vi "Switch Channel.vi"(4 "error in (no error)":errorcluster, 5 "Channel to select":T1(ring), 6 "Card Number":u8=1 min=1 max=5 step=1, 7 "VISA resource in":refnum<visa-resource-name>) -> (0 "error out":errorcluster, 3 "VISA resource out":refnum<visa-resource-name>)   [LabVIEW 2015]
doc: "Switch the multiplexer in the selected card slot to the chosen channel. Designed for use with the HP3488A Switch Unit (5 slots) and the 44476A cards (4 channels)."
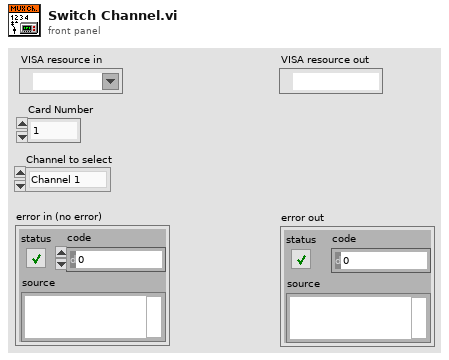
[diagram p1: front panel]
types:
  T1 = enum16{"Channel 1", "Channel 2", "Channel 3", "Channel 4"}
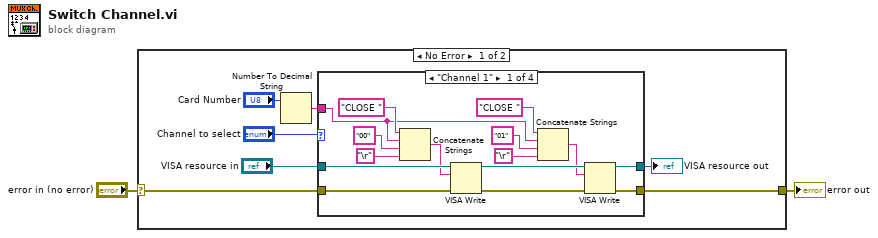
[diagram p0: block diagram]
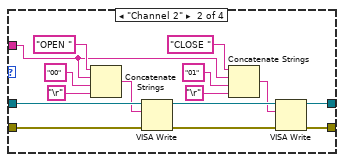
[diagram p2: hidden frame]
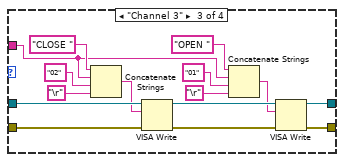
[diagram p3: hidden frame]
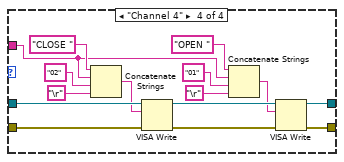
[diagram p4: hidden frame]
diagram:
  n1 = case shown="No Error" "error in (no error)" {
    selector: "error in (no error)" -> [w3 w70]
    tunnel: [w6 w70] -> w2
    frame No Error {
      n2 = Number To Decimal String(number="Card Number") -> (decimal integer string=w4:string)  [unwired: 1 in]
      n3 = case shown="\"Channel 1\"" "Channel to select" {
        tunnel: "VISA resource in" -> [w24 w39 w54 w69]
        tunnel: w3 -> [w23 w38 w53 w68]
        tunnel: [w20 w35 w50 w65] -> w7
        tunnel: [w19 w34 w49 w64] -> w6
        tunnel: w4 -> [w11 w26 w41 w56]
        frame "Channel 1" {
          n4 = Concatenate Strings("CLOSE " ("string"), w11, "00" ("write buffer"), "\r") -> (w16:string)
          n5 = VISA Write(VISA resource name=w24, write buffer=w16, error in (no error)=w23) -> (VISA resource name out=w22:refnum<visa-resource-name>, error out=w21:errorcluster)  [unwired: 1 out]
          n6 = Concatenate Strings("CLOSE " ("string"), w11, "01" ("write buffer"), "\r") -> (w10:string)
          n7 = VISA Write(VISA resource name=w22, write buffer=w10, error in (no error)=w21) -> (VISA resource name out=w20:refnum<visa-resource-name>, error out=w19:errorcluster)  [unwired: 1 out]
        }
        frame "Channel 2" {
          n8 = Concatenate Strings("OPEN " ("string"), w26, "00" ("write buffer"), "\r") -> (w31:string)
          n9 = VISA Write(VISA resource name=w39, write buffer=w31, error in (no error)=w38) -> (VISA resource name out=w37:refnum<visa-resource-name>, error out=w36:errorcluster)  [unwired: 1 out]
          n10 = Concatenate Strings("CLOSE " ("string"), w26, "01" ("write buffer"), "\r") -> (w25:string)
          n11 = VISA Write(VISA resource name=w37, write buffer=w25, error in (no error)=w36) -> (VISA resource name out=w35:refnum<visa-resource-name>, error out=w34:errorcluster)  [unwired: 1 out]
        }
        frame "Channel 3" {
          n12 = Concatenate Strings("CLOSE " ("string"), w41, "02" ("write buffer"), "\r") -> (w46:string)
          n13 = VISA Write(VISA resource name=w54, write buffer=w46, error in (no error)=w53) -> (VISA resource name out=w52:refnum<visa-resource-name>, error out=w51:errorcluster)  [unwired: 1 out]
          n14 = Concatenate Strings("OPEN " ("string"), w41, "01" ("write buffer"), "\r") -> (w40:string)
          n15 = VISA Write(VISA resource name=w52, write buffer=w40, error in (no error)=w51) -> (VISA resource name out=w50:refnum<visa-resource-name>, error out=w49:errorcluster)  [unwired: 1 out]
        }
        frame "Channel 4" {
          n16 = Concatenate Strings("CLOSE " ("string"), w56, "02" ("write buffer"), "\r") -> (w61:string)
          n17 = VISA Write(VISA resource name=w69, write buffer=w61, error in (no error)=w68) -> (VISA resource name out=w67:refnum<visa-resource-name>, error out=w66:errorcluster)  [unwired: 1 out]
          n18 = Concatenate Strings("OPEN " ("string"), w56, "01" ("write buffer"), "\r") -> (w55:string)
          n19 = VISA Write(VISA resource name=w67, write buffer=w55, error in (no error)=w66) -> (VISA resource name out=w65:refnum<visa-resource-name>, error out=w64:errorcluster)  [unwired: 1 out]
        }
      }
      "VISA resource out" <- w7
    }
    frame Error {
    }
  }
  "error out" <- w2
